vi "proceed.vi"(8 "error in (no error)":errorcluster, 11 "ScanModeTS090821Circular2D in":refnum<class "ImagingModeTS090821Circular2D.lvclass">) -> (0 "error out":errorcluster, 2 "sweep finished?":bool, 3 "ScanModeTS090821Circular2D out":refnum<class "ImagingModeTS090821Circular2D.lvclass">)   [LabVIEW 2010, in "ImagingModeTS090821Circular2D.lvclass"]
uses:
  ImagingModeTS090821Circular2D.lvclass
  ImagingModeTS090821Circular2D.lvclass/ImagingModeTS090821Circular2D.ctl
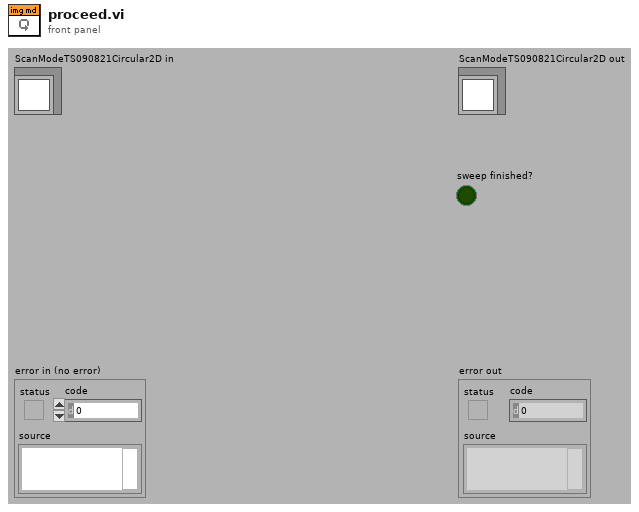
[diagram p1: front panel]
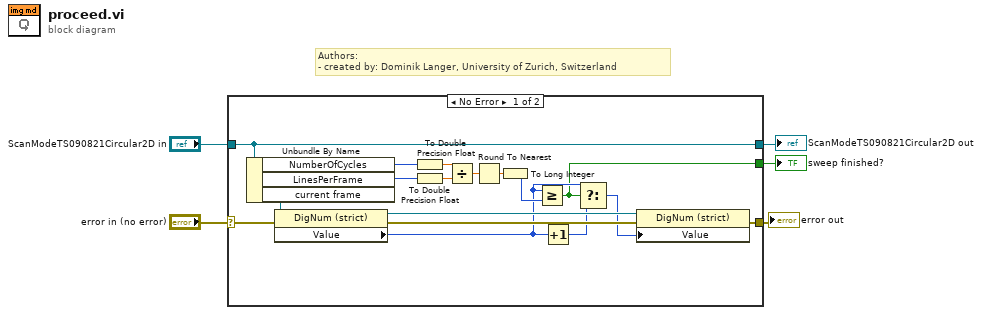
[diagram p0: block diagram]
diagram:
  # "Authors: \n- created by: Dominik Langer, University of Zurich, Switzerland"
  n1 = case shown="No Error" "error in (no error)" {
    selector: "error in (no error)" -> [w22 w23]
    tunnel: "ScanModeTS090821Circular2D in" -> [w18 w24]
    tunnel: [w18 w24] -> w3
    tunnel: [w7 _] -> w2
    tunnel: [w6 w23] -> w1
    frame No Error {
      n2 = Unbundle By Name(w18) -> ("NumberOfCycles"=w17:i32, "LinesPerFrame"=w16:i32, "current frame"=w21:refnum<vi>)
      n3 = property class="DigNum (strict)"(reference=w21, error in=w22) -> (reference out=w19:refnum<vi>, error out=w20:errorcluster, "Value"=w9:i32)
      n4 = To Double Precision Float(number=w17) -> (double precision float=w15:dbl)
      n5 = To Double Precision Float(number=w16) -> (double precision float=w14:dbl)
      n6 = Divide(x=w15, y=w14) -> (x/y=w13:dbl)
      n7 = Round To Nearest(number=w13) -> (nearest integer value=w12:dbl)
      n8 = To Long Integer(number=w12) -> (32bit integer=w11:i32)
      n9 = Greater Or Equal?(x=w9, y=w11) -> (x >= y?=w7:bool)
      n10 = Increment(x=w9) -> (x+1=w10:i32)
      n11 = Select(t=w9, s=w7, f=w10) -> (s? t:f=w8:i32)
      n12 = property class="DigNum (strict)"(reference=w19, error in=w20, "Value"=w8) -> (error out=w6:errorcluster)  [unwired: 1 out]
    }
    frame Error {
    }
  }
  "error out" <- w1
  "ScanModeTS090821Circular2D out" <- w3
  "sweep finished?" <- w2
